vi "Save_Destination_Type.vi"(8 "error in (no error)":errorcluster, 9 "index":i32, 10 "buildObject":T1, 11 "AB_Dest_App in":refnum<class "AB_Dest_LegacyApp.lvclass">) -> (0 "error out":errorcluster, 3 "AB_Dest_App out":refnum<class "AB_Dest_LegacyApp.lvclass">)   [LabVIEW 2020, in "AB_Dest_LegacyApp.lvclass"]
uses:
  <vilib>/AppBuilder/AB_Classes/Destination/Dest_LegacyApplication/AB_Dest_LegacyApp.lvclass
  <resource>/Framework/Providers/API/ItemRef.ctl
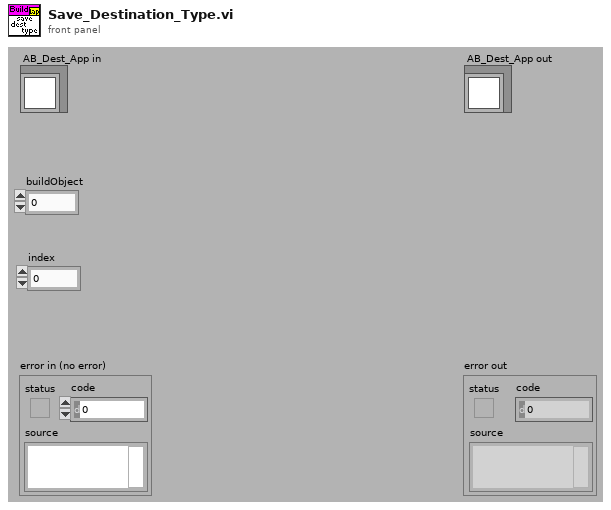
[diagram p1: front panel]
types:
  T1 = typedef "ItemRef.ctl" = u64
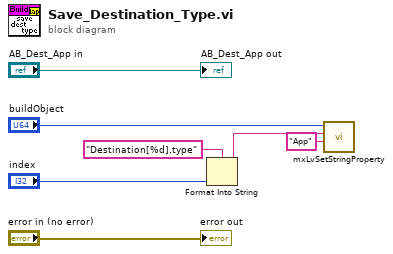
[diagram p0: block diagram]
diagram:
  n1 = Format Into String(format string="Destination[%d].type", "index") -> (resulting string=w4:string)  [unwired: 2 in, 1 out]
  n2 = call <resource>:"mxLvSetStringProperty.vi"("Value (\"\")"="App" ("Value (\"\")"), "Tag"=w4, "Item"="buildObject") -> ()  [unwired: 2 in, 7 out]
  "error out" <- "error in (no error)"
  "AB_Dest_App out" <- "AB_Dest_App in"
